vi "Get Monitoring CD ports.vi"(8 "Error In":errorcluster, 11 "Device Item Ref in":T1 format="%.0x") -> (0 "Error Out":errorcluster, 1 "Referenced NI-XNET Port Item Paths":string[](array[string]), 2 "CD Port Refs":T1[](array[typedef]) format="%.0x", 3 "Device Item Ref out":T1 format="%.0x")   [LabVIEW 2017, in "NI-XNET Monitor System Explorer.lvlib"]
uses:
  NI-XNET Monitor System Explorer.lvlib
  <vilib>/NI Veristand/Custom Device API/Custom Device Item Ref.ctl
  <vilib>/NI Veristand/Custom Device Tools/Custom Device Utility Library/Search Direction.ctl
  Shared/Constants.vi
  <vilib>/NI Veristand/Custom Device Tools/Custom Device Utility Library/NI VeriStand - Search for Item by GUID.vi
  <vilib>/NI Veristand/Custom Device Tools/Custom Device Utility Library/NI VeriStand - Search for All Items by GUID.vi
  <vilib>/NI Veristand/Custom Device API/Get Item Property (String).vi
  <vilib>/NI VeriStand/Custom Device Tools/Custom Device Utility Library/Custom Device Utility Library.lvlib
  Shared/NI-XNET Monitor Shared.lvlib
  <vilib>/NI Veristand/Custom Device API/Custom Device API.lvlib
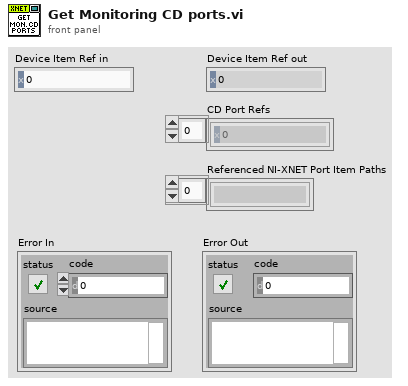
[diagram p1: front panel]
types:
  T1 = typedef "Custom Device API.lvlib/Custom Device Item Ref.ctl" = u64
  T2 = typedef "Custom Device Utility Library.lvlib/Search Direction.ctl" = enum16{"Down", "Up"}
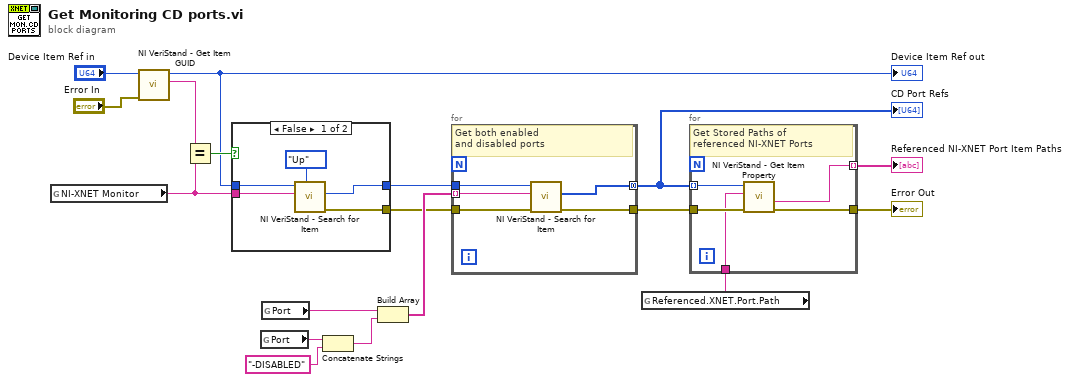
[diagram p0: block diagram]
diagram:
  n1 = global read "Constants.vi" "NI-XNET Monitor"() -> (w10:string)
  n2 = call <vilib>:"NI VeriStand - Get Item GUID.vi"("error in (no error)"="Error In", "Item Ref in"="Device Item Ref in") -> ("GUID"=w11:string, "Item Ref out"=w3:T1)  [unwired: 7 in, 1 out]
  "Device Item Ref out" <- w3
  n3 = Equal?(x=w11, y=w10) -> (x = y?=w9:bool)
  n4 = case shown="False" w9 {
    tunnel: [w22 _] -> w7
    tunnel: [w21 w24] -> w8
    tunnel: w3 -> [w20 w24]
    tunnel: w10 -> [w19 _]
    frame False {
      n5 = call-poly <vilib>:"NI VeriStand - Search for Item.vi"("Direction (Down)"=Search_Direction."Up", "Item GUID"=w19, "Section Ref in"=w20) -> ("error out"=w22:errorcluster, "Item Ref"=w21:T1)  [unwired: 5 in, 2 out]
    }
    frame True {
    }
  }
  n6 = global read "Constants.vi" "Port"() -> (w16:string)
  n7 = global read "Constants.vi" "Port"() -> (w14:string)
  n8 = Concatenate Strings(w16, "-DISABLED" ("regular expression")) -> (w13:string)
  n9 = Build Array(w14, w13) -> (w12:string[])
  n10 = for {
    tunnel: w8 -> [w29]
    tunnel: w7 -> [w28]
    tunnel: w12 -> [w27] mode=indexing
    tunnel: [w26] -> w5 mode=concatenating
    tunnel: [w25] -> w2
    # "Get both enabled\nand disabled ports"
    n11 = call-poly <vilib>:"NI VeriStand - Search for Item.vi"("error in"=w28, "Item GUID"=w27, "Section Ref in"=w29) -> ("error out"=w25:errorcluster, "Item Refs"=w26:T1[])  [unwired: 5 in, 2 out]
  }
  "CD Port Refs" <- w5
  n12 = global read "Constants.vi" "Referenced.XNET.Port.Path"() -> (w1:string)
  n13 = for {
    tunnel: w5 -> [w34] mode=indexing
    tunnel: [w32] -> w18
    tunnel: [w31] -> w17 mode=indexing
    tunnel: w2 -> [w33]
    tunnel: w1 -> [w30]
    # "Get Stored Paths of\nreferenced NI-XNET Ports"
    n14 = call-poly <vilib>:"NI VeriStand - Get Item Property.vi"("error in (no error)"=w33, "Property Name"=w30, "Item Ref in"=w34) -> ("error out"=w32:errorcluster, "Value"=w31:string)  [unwired: 5 in, 2 out]
  }
  "Error Out" <- w18
  "Referenced NI-XNET Port Item Paths" <- w17
